vi "SPC_get_sequencer_state.vi"(8 "Error In":errorcluster, 10 "Module No":i16 min=0 max=7 step=1, 11 "DLL Path":path) -> (0 "Error Out":errorcluster, 2 "Module No":i16 min=0 max=7 step=1, 3 "DLL Path":path, 4 "State Value":i16 format="%.0x", 5 "Status":T1)   [LabVIEW 2023]
doc: "The procedure is used to get the current state of the sequencer status bits on SPC module 'mod_no'. The sequencer status bits are defined in the spcm_def.h file:\nSPC_SEQ_ENABLE 0x1 sequencer is enabled\nSPC_SEQ_RUNNING 0x2 sequencer is running\nonly for SPC6x0/13x/15x/160 modules\nSPC_SEQ_GAP_BANK 0x4 sequencer is waiting for other bank to be armed\n\ninfo@becker-hickl.com"
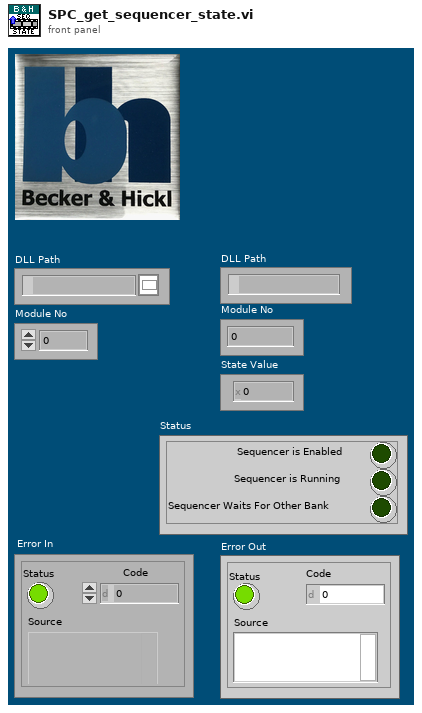
[diagram p1: front panel]
types:
  T1 = cluster{"Sequencer is Enabled":bool, "Sequencer is Running":bool, "Sequencer Waits For Other Bank":bool}
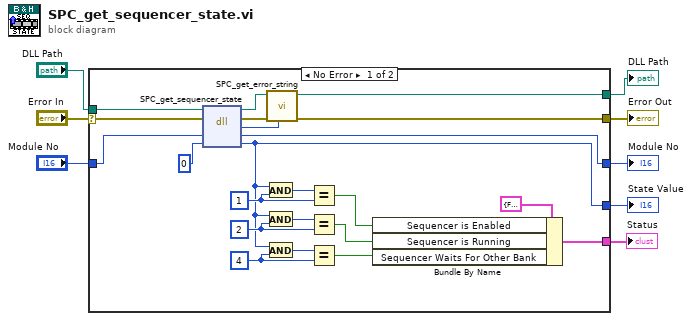
[diagram p0: block diagram]
diagram:
  n1 = case shown="No Error" "Error In" {
    selector: "Error In" -> [w29 w32]
    tunnel: "DLL Path" -> [w30 w33]
    tunnel: [w27 w32] -> w6
    tunnel: [w24 w33] -> w5
    tunnel: [w15 _] -> w4
    tunnel: "Module No" -> [w23 w31]
    tunnel: [w22 w31] -> w2
    tunnel: [w10 _] -> w1
    frame No Error {
      w17 = i16 4
      w16 = i16 2
      w19 = i16 1
      n2 = dll-call lib="D:/spcm/lib/lab_view/lv10.0/spcm32.dll" fn="SPC_get_sequencer_state"(path in=w30, error in=w29, "mod_no"=w23, "state"=i16 0 ("Last State Value")) -> (path out=w25:path, error out=w28:errorcluster, "return type"=w26:i16, "mod_no"=w22:i16, "state"=w15:i16)  [unwired: 1 in]
      n3 = And(x=w15, y=w19) -> (x .and. y?=w20:i16)
      n4 = And(x=w15, y=w16) -> (x .and. y?=w12:i16)
      n5 = And(x=w15, y=w17) -> (x .and. y?=w11:i16)
      n6 = call "SPC_get_error_string.vi"("ErrorID"=w26, "Error In"=w28, "DLL Path"=w25) -> ("Error Out"=w27:errorcluster, "DLL Path"=w24:path)  [unwired: 6 in, 1 out]
      n7 = Equal?(x=w20, y=w19) -> (x = y?=w18:bool)
      n8 = Equal?(x=w12, y=w16) -> (x = y?=w13:bool)
      n9 = Equal?(x=w11, y=w17) -> (x = y?=w14:bool)
      n10 = Bundle By Name(cluster=T1 {"Sequencer is Enabled"=FALSE, "Sequencer is Running"=FALSE, "Sequencer Waits For Other Bank"=FALSE} ("Status"), "Sequencer is Enabled"=w18, "Sequencer is Running"=w13, "Sequencer Waits For Other Bank"=w14) -> (w10:T1)
    }
    frame Error {
    }
  }
  "Error Out" <- w6
  "DLL Path" <- w5
  "State Value" <- w4
  "Module No" <- w2
  "Status" <- w1
